vi "Read TDMS File _0.vi"() -> ()   [LabVIEW 2012]
doc: "Reads a TDMS (Technical Data Management Streaming) file."
panel:
  out "Waveform Graph":waveform(dbl)[](graph)
  # "This example reads measured data from a TDMS file."
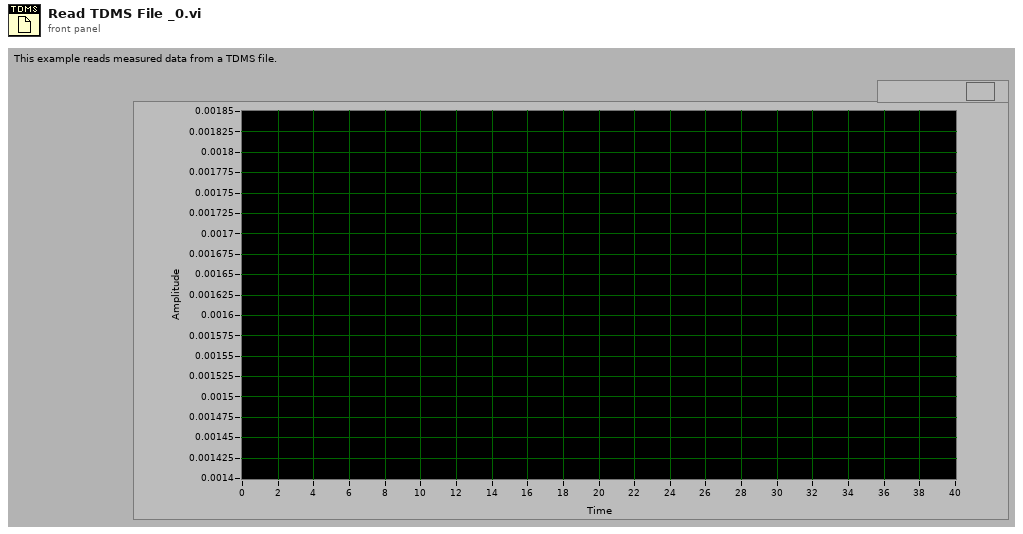
[diagram p1: front panel]
types:
  T1 = enum16{"open", "open or create", "create or replace", "create", "open (read-only)"}
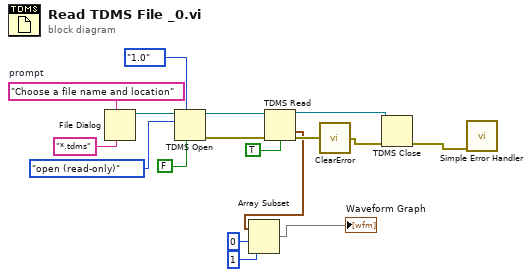
[diagram p0: block diagram]
diagram:
  w14 = "Choose a file name and location"  # prompt
  n1 = File Dialog(6:"*.tdms" ("pattern (all files)"), 7:w14) -> (3:w13:path)  [unwired: 1 in, 7 out]
  n2 = TDMS Open(6:FALSE ("disable buffering (T)"), 7:enum16{"1.0", "2.0"}."1.0" ("file format version (2.0)"), 10:T1."open (read-only)" ("operation"), 11:w13) -> (0:w9:errorcluster, 3:w10:refnum<k34>)  [unwired: 2 in]
  n3 = TDMS Read(0:w10, 11:w9, 13:TRUE ("return channels in file order? (F)")) -> (4:w16:refnum<k34>, 10:w4:waveform(dbl)[], 15:w6:errorcluster)  [unwired: 5 in, 3 out]
  n4 = Array Subset(array=w4, index=0, length=1) -> (→"Waveform Graph":waveform(dbl)[])
  n5 = call <vilib>:"ClearError.vi"("error in (no error)"=w6) -> ("error out"=w15:errorcluster)
  n6 = TDMS Close(8:w15, 11:w16) -> (0:w17:errorcluster)  [unwired: 1 out]
  n7 = call <vilib>:"Simple Error Handler.vi"("error in (no error)"=w17) -> ()  [unwired: 1 in, 8 out]
